vi "TimeInterpBoolean_AddSample.vi"(9 "Value":bool, 10 "TimeStamp":dbl, 11 "in TimeInterpBoolean":T1) -> (0 "Error":bool, 3 "out TimeInterpBoolean":T1)   [LabVIEW 2019, in "Trajectory_Library.lvlib"]
doc: "Add a sample to the buffer.\n \nInputs:\n - In TimeInterpBoolean -- Time Interp data cluster \n - Time -- The time stamp of the sample (seconds)\n - Value -- The boolean value\n\nOutputs:\n - out TimeInterpBoolean -- Updated Time Interp data cluster"
uses:
  Trajectory_Library.lvlib
  TypeDef/TIME_INTERPOLATABLE_BOOLEAN.ctl
  <vilib>/gmath/NI_Gmath.lvlib
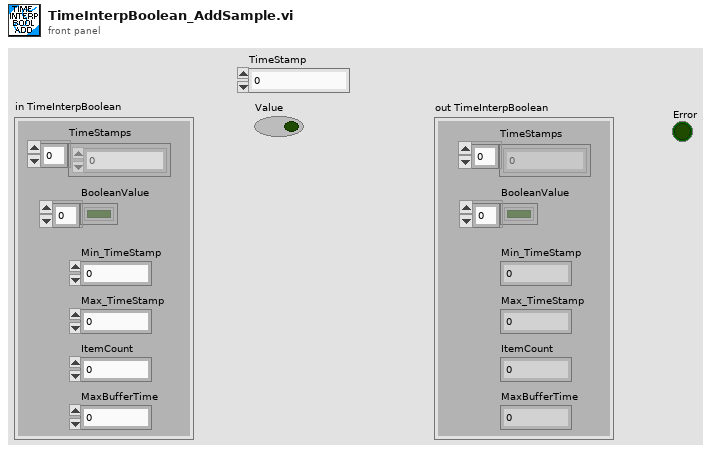
[diagram p1: front panel]
types:
  T1 = typedef "Trajectory_Library.lvlib/TIME_INTERPOLATABLE_BOOLEAN.ctl" = cluster{"TimeStamps":dbl[], "BooleanValue":bool[], "Min_TimeStamp":dbl, "Max_TimeStamp":dbl, "ItemCount":i32, "MaxBufferTime":dbl}
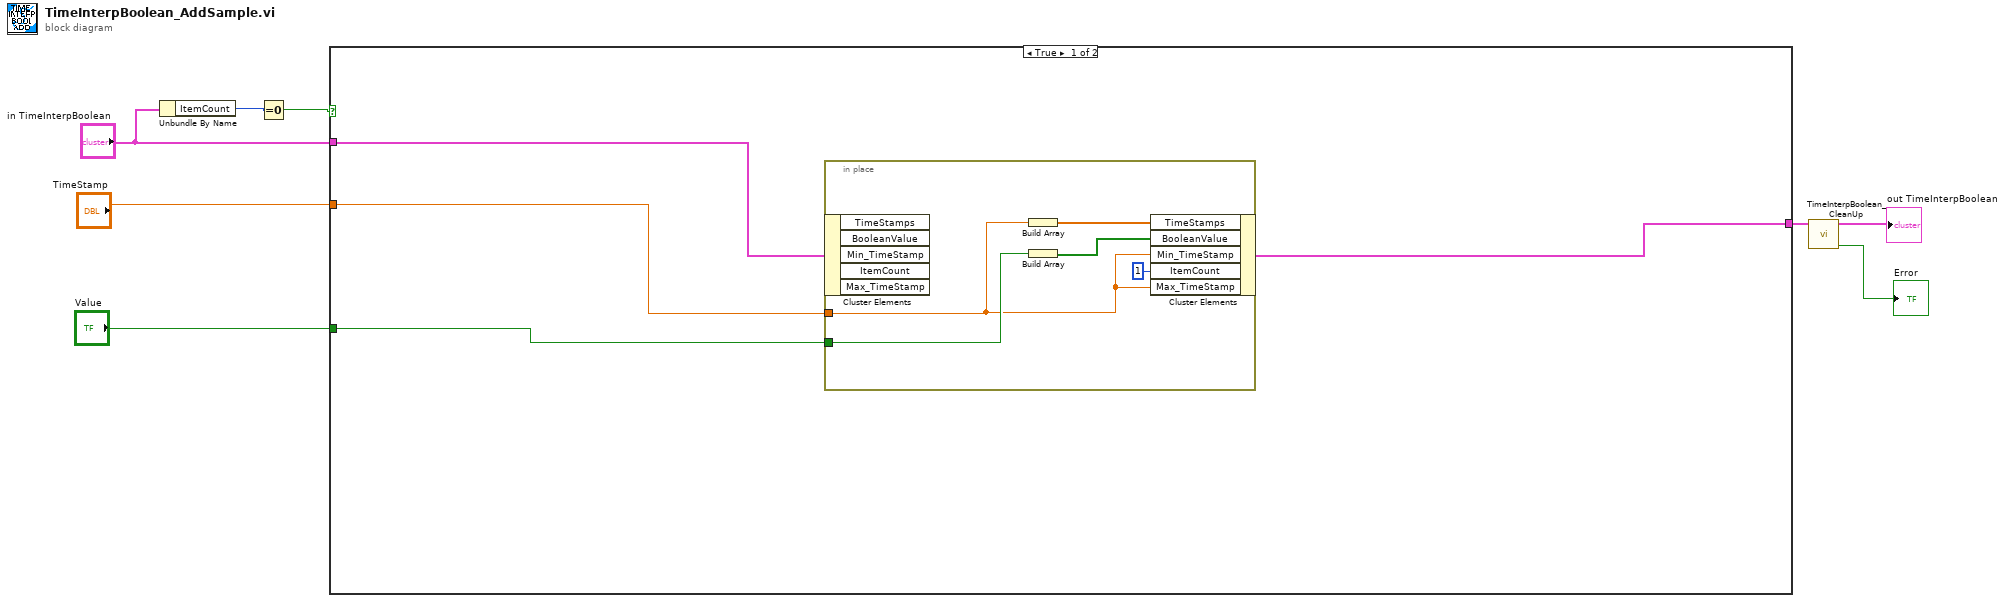
[diagram p0: block diagram]
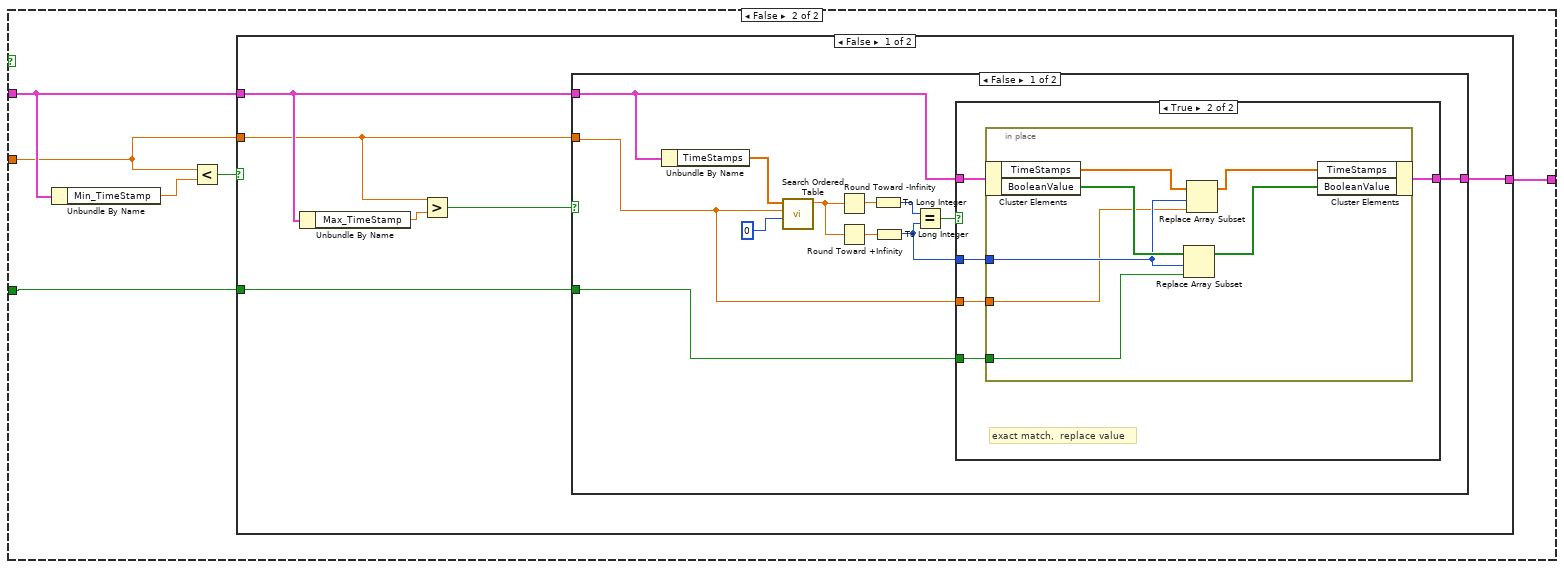
[diagram p2: hidden frame]
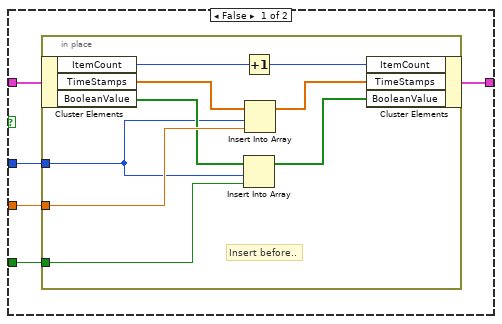
[diagram p3: hidden frame]
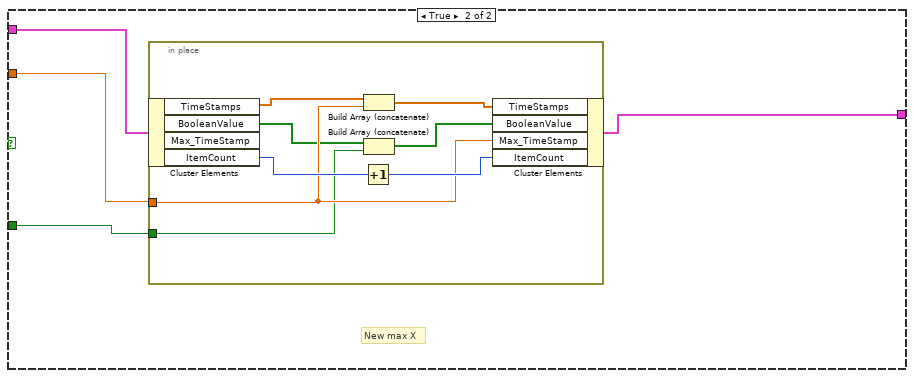
[diagram p4: hidden frame]
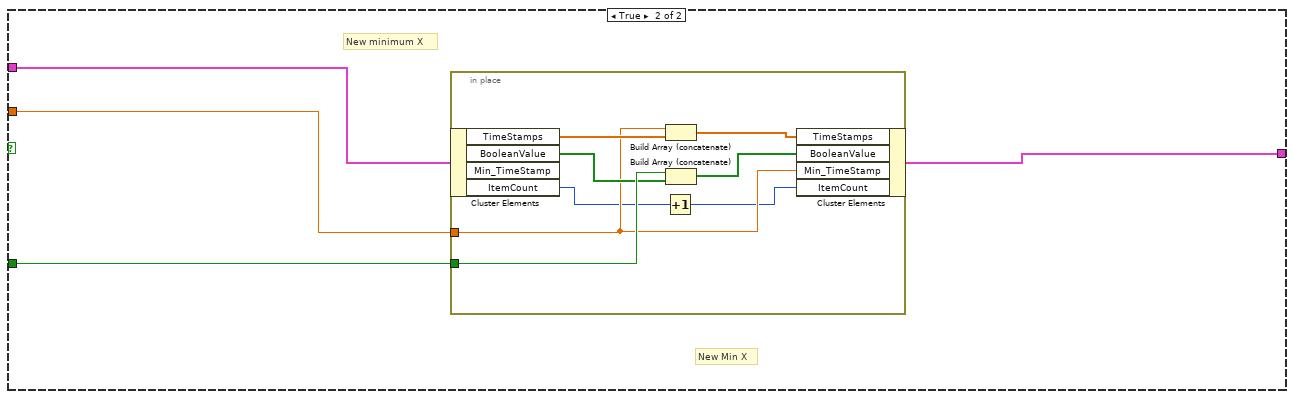
[diagram p5: hidden frame]
diagram:
  n1 = Unbundle By Name("in TimeInterpBoolean") -> ("ItemCount"=w2:i32)
  n2 = Equal To 0?(x=w2) -> (x = 0?=w1:bool)
  n3 = case shown="True" w1 {
    tunnel: "in TimeInterpBoolean" -> [w12 w21]
    tunnel: "TimeStamp" -> [w11 w20]
    tunnel: "Value" -> [w10 w19]
    tunnel: [w9 w18] -> w6
    frame True {
      n4 = in-place {
        in-place-border: w11 -> [w14]
        in-place-border: w10 -> [w17]
        n5 = in-place-cluster #1(w12) -> ()  [unwired: 5 out]
        n6 = Build Array(w14) -> (w16:dbl[])
        n7 = Build Array(w17) -> (w15:bool[])
        n8 = in-place-cluster #1("TimeStamps"=w16, "BooleanValue"=w15, "Min_TimeStamp"=w14, "ItemCount"=1, "Max_TimeStamp"=w14) -> (w9:T1)
      }
    }
    frame False {
      n9 = Unbundle By Name(w21) -> ("Min_TimeStamp"=w23:dbl)
      n10 = Less?(x=w20, y=w23) -> (x < y?=w22:bool)
      n11 = case shown="False" w22 {
        tunnel: w21 -> [w28 w83]
        tunnel: w20 -> [w26 w82]
        tunnel: w19 -> [w25 w81]
        tunnel: [w27 w80] -> w18
        frame False {
          n12 = Unbundle By Name(w28) -> ("Max_TimeStamp"=w29:dbl)
          n13 = Greater?(x=w26, y=w29) -> (0:w24:bool)
          n14 = case shown="False" w24 {
            tunnel: w28 -> [w34 w71]
            tunnel: [w30 w70] -> w27
            tunnel: w26 -> [w32 w69]
            tunnel: w25 -> [w31 w68]
            frame False {
              n15 = Unbundle By Name(w34) -> ("TimeStamps"=w40:dbl[])
              n16 = call <vilib>:"Search Ordered Table.vi"("starting index"=0, "x value"=w32, "ordered x array"=w40) -> ("fractional index"=w39:dbl)  [unwired: 8 in]
              n17 = Round Toward -Infinity(1:w39) -> (0:w37:dbl)
              n18 = Round Toward +Infinity(x=w39) -> (ceil(x): smallest int >= x=w38:dbl)
              n19 = To Long Integer(number=w37) -> (32bit integer=w36:i32)
              n20 = To Long Integer(number=w38) -> (32bit integer=w33:i32)
              n21 = Equal?(x=w36, y=w33) -> (x = y?=w35:bool)
              n22 = case shown="True" w35 {
                tunnel: w34 -> [w43 w60]
                tunnel: w33 -> [w46 w59]
                tunnel: w32 -> [w45 w58]
                tunnel: w31 -> [w44 w57]
                tunnel: [w42 w56] -> w30
                frame False {
                  n23 = in-place {
                    in-place-border: w46 -> [w50]
                    in-place-border: w45 -> [w52]
                    in-place-border: w44 -> [w49]
                    # "Insert before.."
                    n24 = in-place-cluster #2(w43) -> ("ItemCount"=w55:i32, "TimeStamps"=w53:dbl[], "BooleanValue"=w51:bool[])
                    n25 = Increment(x=w55) -> (x+1=w54:i32)
                    n26 = Insert Into Array(array=w51, index=w50, new element=w49) -> (w47:bool[])
                    n27 = Insert Into Array(array=w53, index=w50, new element=w52) -> (w48:dbl[])
                    n28 = in-place-cluster #2("ItemCount"=w54, "TimeStamps"=w48, "BooleanValue"=w47) -> (w42:T1)
                  }
                }
                frame True {
                  # "exact match,  replace value"
                  n29 = in-place {
                    in-place-border: w59 -> [w65]
                    in-place-border: w58 -> [w64]
                    in-place-border: w57 -> [w63]
                    n30 = in-place-cluster #3(w60) -> ("TimeStamps"=w67:dbl[], "BooleanValue"=w66:bool[])
                    n31 = Replace Array Subset(array=w66, new element=w63, index=w65) -> (w61:bool[])
                    n32 = Replace Array Subset(array=w67, new element=w64, index=w65) -> (w62:dbl[])
                    n33 = in-place-cluster #3("TimeStamps"=w62, "BooleanValue"=w61) -> (w56:T1)
                  }
                }
              }
            }
            frame True {
              # "New max X"
              n34 = in-place {
                in-place-border: w69 -> [w75]
                in-place-border: w68 -> [w72]
                n35 = in-place-cluster #4(w71) -> ("TimeStamps"=w74:dbl[], "BooleanValue"=w73:bool[], "ItemCount"=w77:i32)  [unwired: 1 out]
                n36 = Increment(x=w77) -> (x+1=w76:i32)
                n37 = Build Array (concatenate)(w74, w75) -> (w79:dbl[])
                n38 = Build Array (concatenate)(w73, w72) -> (w78:bool[])
                n39 = in-place-cluster #4("TimeStamps"=w79, "BooleanValue"=w78, "Max_TimeStamp"=w75, "ItemCount"=w76) -> (w70:T1)
              }
            }
          }
        }
        frame True {
          # "New Min X"
          # "New minimum X"
          n40 = in-place {
            in-place-border: w82 -> [w86]
            in-place-border: w81 -> [w91]
            n41 = in-place-cluster #5(w83) -> ("TimeStamps"=w90:dbl[], "BooleanValue"=w87:bool[], "ItemCount"=w85:i32)  [unwired: 1 out]
            n42 = Increment(x=w85) -> (x+1=w84:i32)
            n43 = Build Array (concatenate)(w86, w90) -> (w89:dbl[])
            n44 = Build Array (concatenate)(w91, w87) -> (w88:bool[])
            n45 = in-place-cluster #5("TimeStamps"=w89, "BooleanValue"=w88, "Min_TimeStamp"=w86, "ItemCount"=w84) -> (w80:T1)
          }
        }
      }
    }
  }
  n46 = call "TimeInterpBoolean_CleanUp.vi"("in TimeInterpBoolean"=w6) -> ("Error"=→"Error":bool, "out TimeInterpBoolean"=→"out TimeInterpBoolean":T1)  [unwired: 9 in]
